vi "Strings and Formats.vi"(0 "TTLControl in":refnum<class "TTLController.lvclass">, 11 "error in (no error)":errorcluster) -> (4 "TTLControl out":refnum<class "TTLController.lvclass">, 8 "Strings[] and Formats[]":cluster{"Strings":string[], "Formats":string[]}, 15 "error out":errorcluster)   [LabVIEW 2015, in "TTLController.lvclass"]
uses:
  TTLController.lvclass
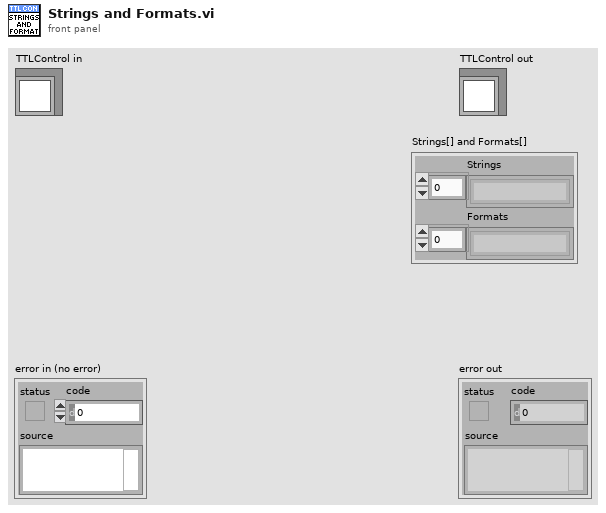
[diagram p1: front panel]
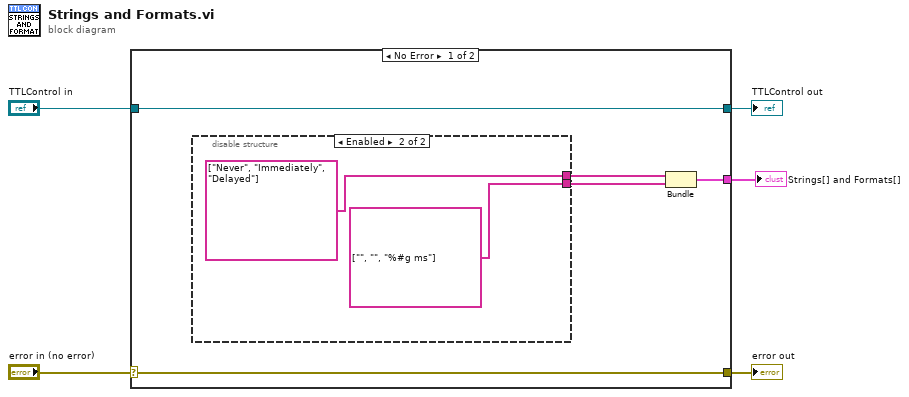
[diagram p0: block diagram]
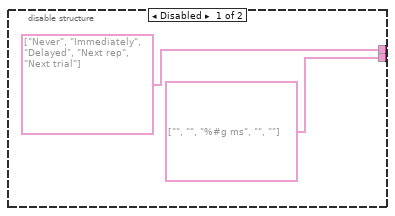
[diagram p2: hidden frame]
diagram:
  n1 = case shown="No Error" "error in (no error)" {
    selector: "error in (no error)" -> [w9 w16]
    tunnel: [w9 w16] -> w4
    tunnel: [w10 w15] -> w2
    tunnel: "TTLControl in" -> [w10 w15]
    tunnel: [w6 _] -> w1
    frame No Error {
      n2 = disable-structure shown="Enabled" {
        disable-tunnel: [string[] ["Never", "Immediately", "Delayed", "Next rep", "Next trial"] ("Strings") string[] ["Never", "Immediately", "Delayed"] ("Strings")] -> w8
        disable-tunnel: [string[] ["", "", "%#g ms", "", ""] ("Strings") string[] ["", "", "%#g ms"] ("Strings")] -> w7
        frame Disabled {
        }
        frame Enabled {
        }
      }
      n3 = Bundle("Strings"=w8, "Strings"=w7) -> (w6:cluster{"Strings":string[], "Strings":string[]})  [unwired: 1 in]
    }
    frame Error {
    }
  }
  "error out" <- w4
  "TTLControl out" <- w2
  "Strings[] and Formats[]" <- w1
